vi "get path to CoreEngine dll.vi"() -> (8 "path to wavekit library":path, 12 "Release/Debug":string)   [LabVIEW 2020]
uses:
  <vilib>/registry/registry.llb/Registry RtKey.ctl
  <vilib>/registry/registry.llb/Registry SAM.ctl
  <vilib>/registry/registry.llb/Read Registry Value Simple STR.vi
panel:
  in  "error in (no error)":errorcluster
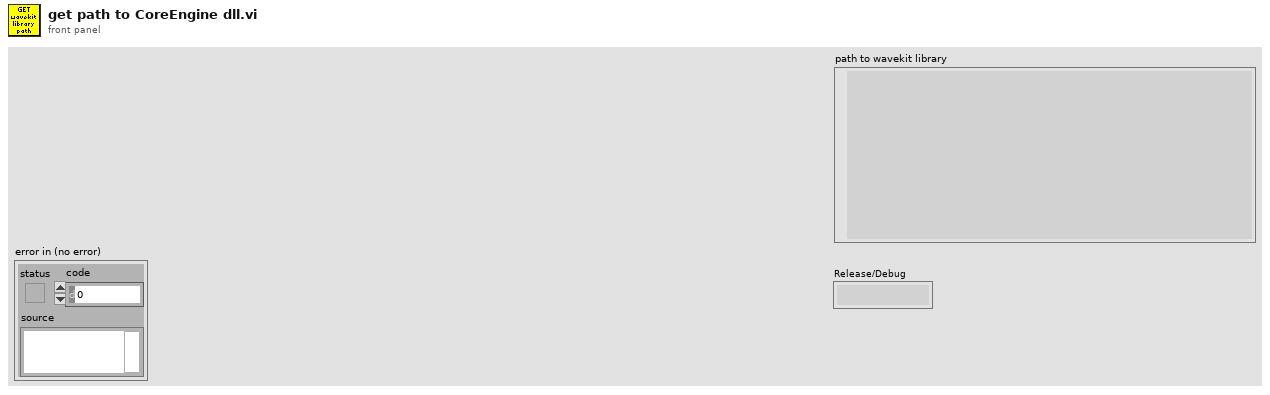
[diagram p1: front panel]
types:
  T1 = typedef "Registry SAM.ctl" = enum32{"KEY_QUERY_VALUE", "KEY_SET_VALUE", "KEY_CREATE_SUB_KEY", "KEY_ENUMERATE_SUB_KEYS", "KEY_NOTIFY", "KEY_CREATE_LINK", "KEY_READ", "KEY_WRITE", "KEY_ALL_ACCESS", "KEY_READ | KEY_WRITE"}
  T2 = typedef "Registry RtKey.ctl" = enum32{"HKEY_CLASSES_ROOT", "HKEY_CURRENT_USER", "HKEY_LOCAL_MACHINE", "HKEY_USERS", "HKEY_PERFORMANCE_DATA", "HKEY_CURRENT_CONFIG", "HKEY_DYN_DATA"}
  T3 = enum32{"invalid app kind", "Development System", "Run Time System", "Student Edition", "Embedded LabVIEW", "Evaluation", "Custom"}
  T4 = typedef "Registry refnum.ctl" = refnum<k1>
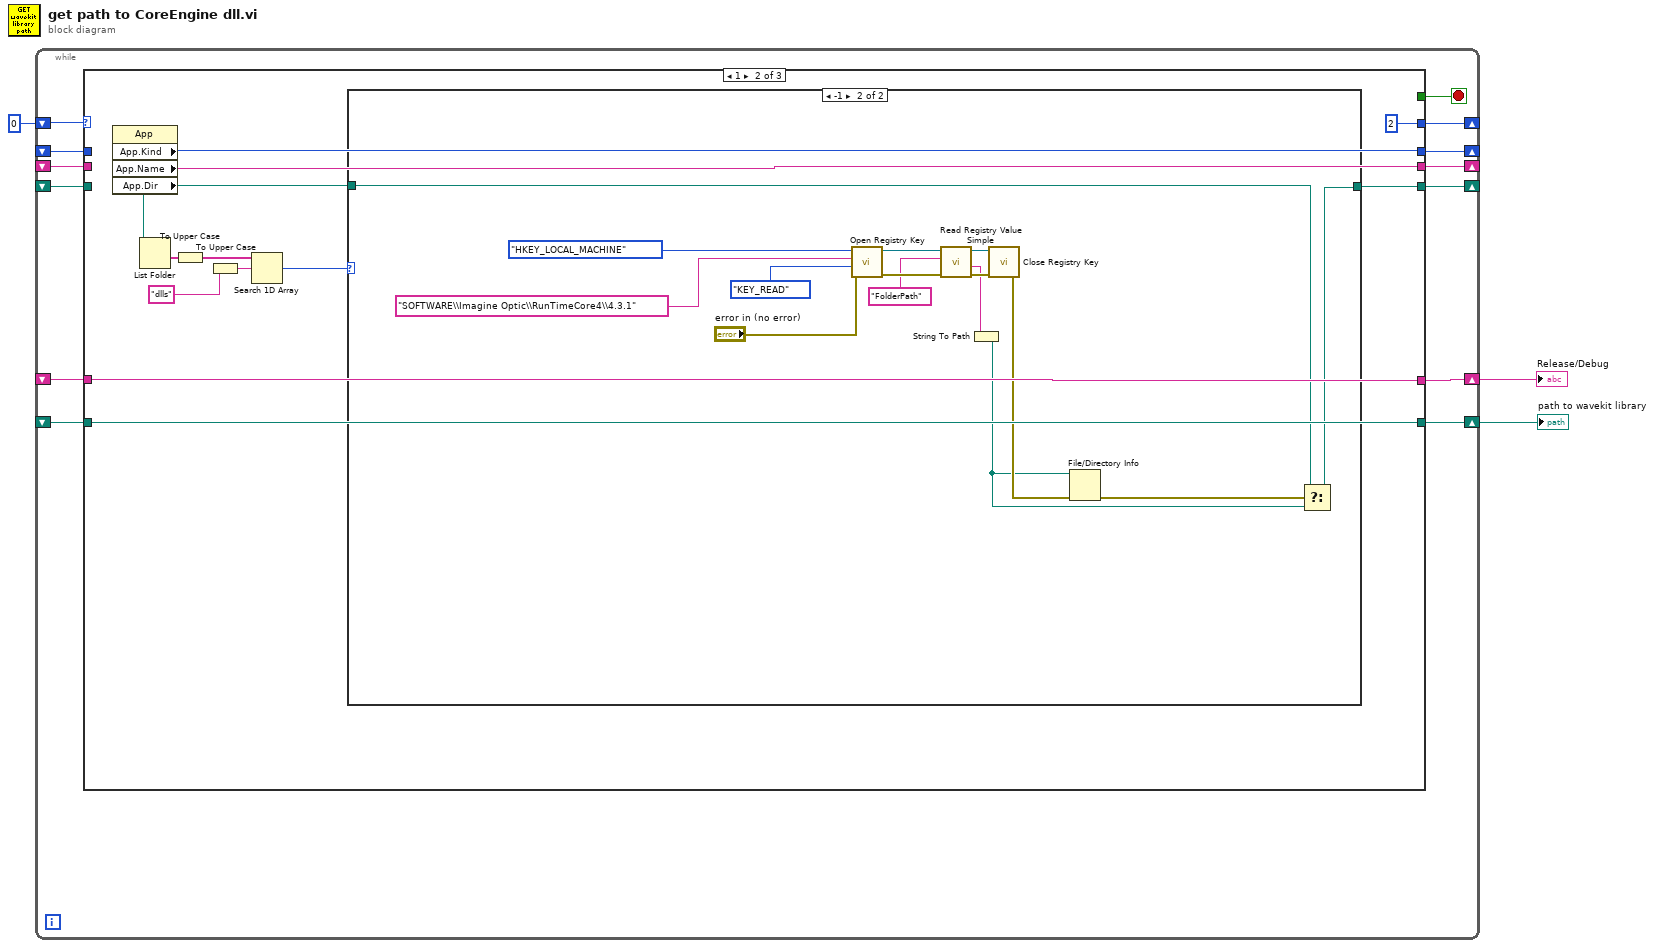
[diagram p0: block diagram]
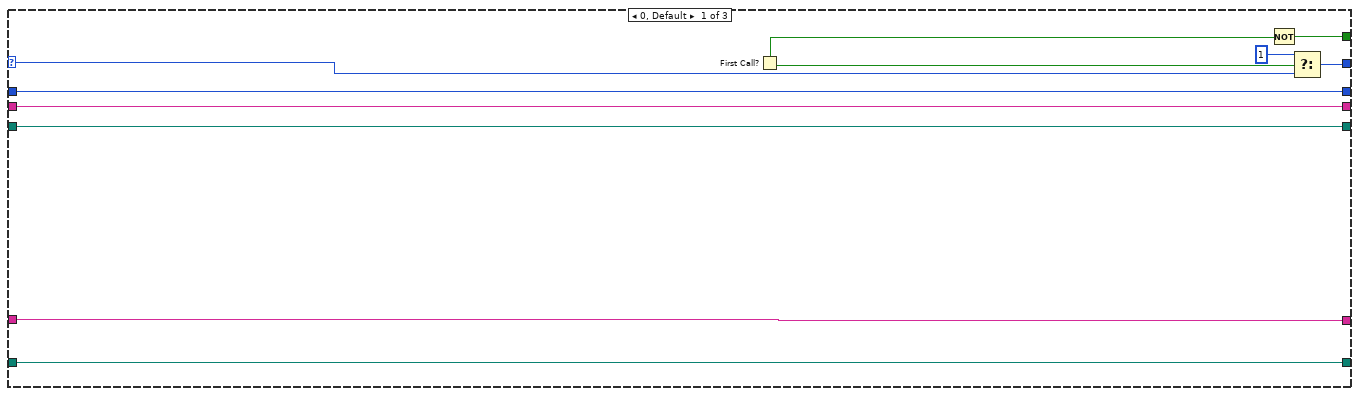
[diagram p2: hidden frame]
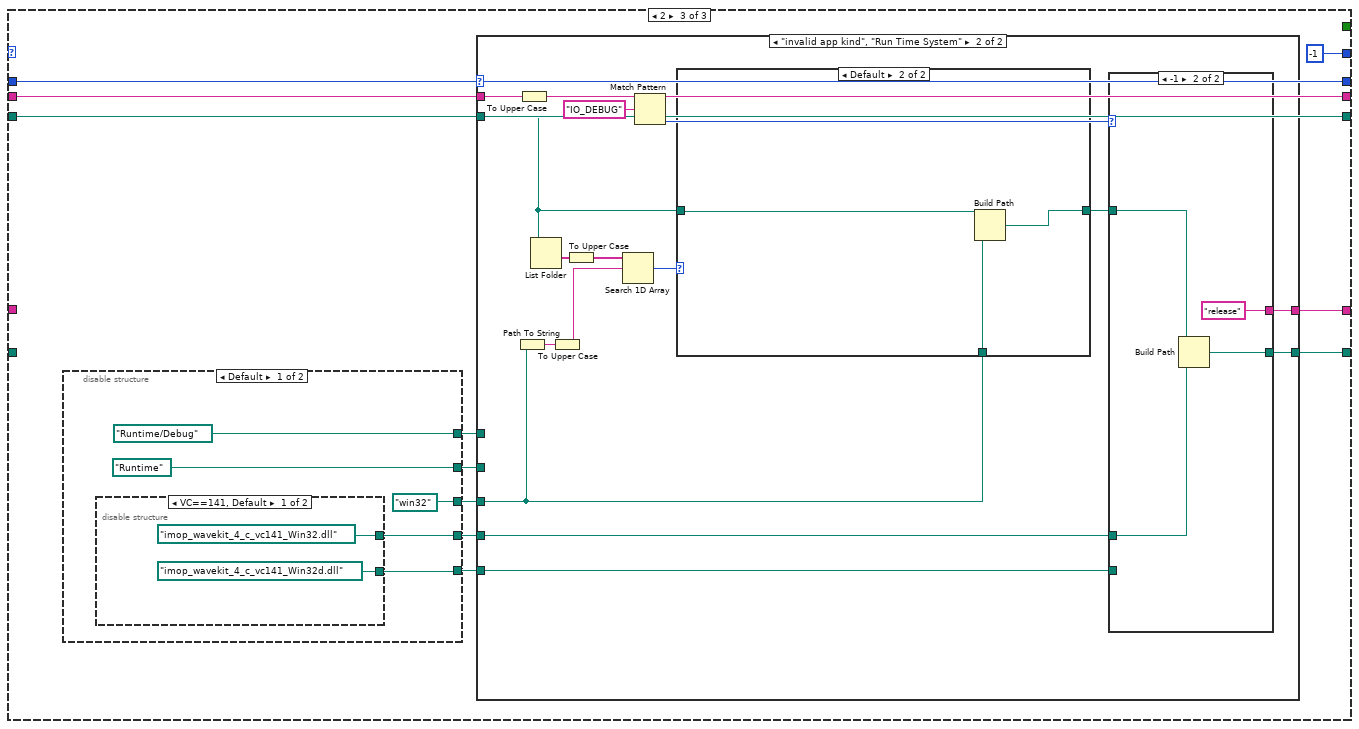
[diagram p4: hidden frame]
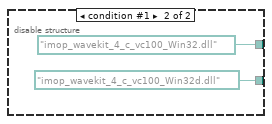
[diagram p5: hidden frame]
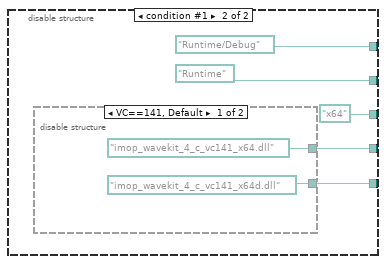
[diagram p6: hidden frame]
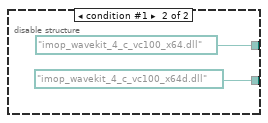
[diagram p7: hidden frame]
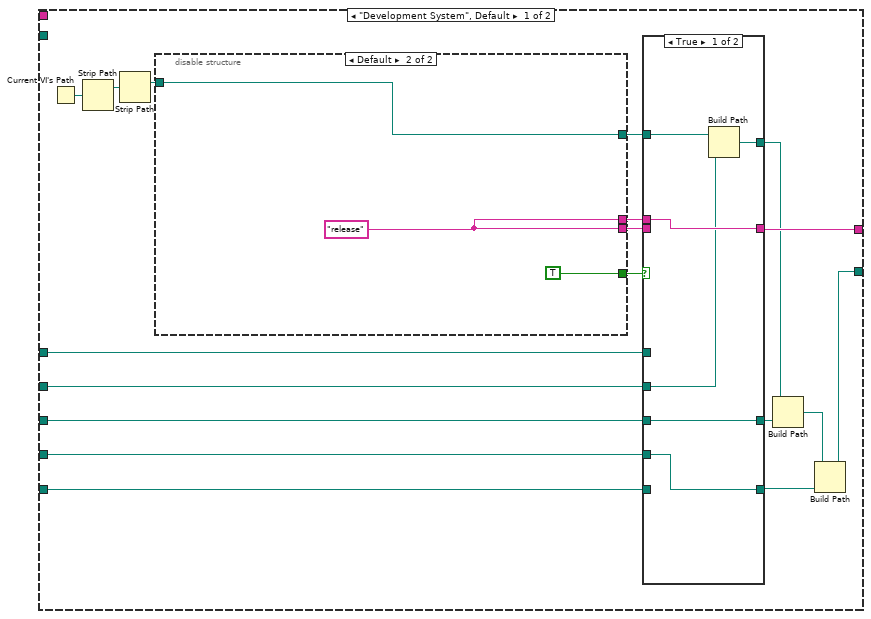
[diagram p8: hidden frame]
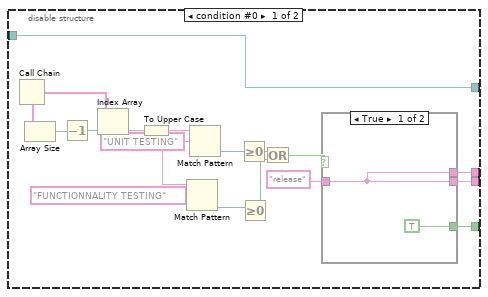
[diagram p9: hidden frame]
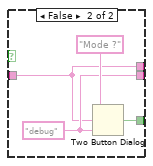
[diagram p10: hidden frame]
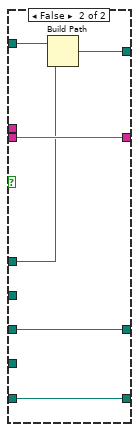
[diagram p11: hidden frame]
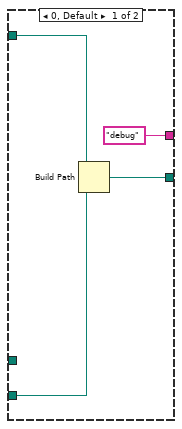
[diagram p12: hidden frame]
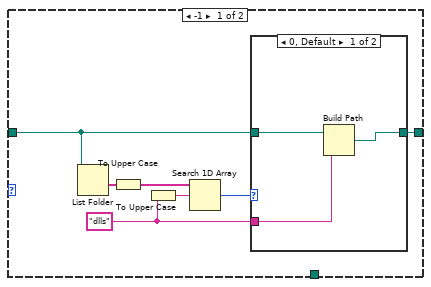
[diagram p13: hidden frame]
diagram:
  n1 = while {
    shift-right: [w14] -> _
    shift-left: 0 -> [w15]
    shift-right: [w12] -> _
    shift-left: _ -> [w9]
    shift-right: [w11] -> _
    shift-left: _ -> [w10]
    shift-right: [w16] -> w3
    shift-left: _ -> [w8]
    shift-right: [w7] -> w1
    shift-left: _ -> [w6]
    shift-right: [w5] -> _
    shift-left: _ -> [w4]
    stop <- w13 stop-if-true
    n2 = case shown="1" w15 {
      selector: w15 -> [w23 _ _]
      tunnel: [w19 w35 w65] -> w16
      tunnel: [w26 2 -1] -> w14
      tunnel: [w22 _ _] -> w13
      tunnel: [w21 w37 w63] -> w12
      tunnel: [w20 w36 w62] -> w11
      tunnel: w10 -> [w20 _ w62]
      tunnel: w9 -> [w21 _ w63]
      tunnel: w8 -> [w19 w35 _]
      tunnel: [w18 w34 w61] -> w7
      tunnel: w6 -> [w18 w34 _]
      tunnel: [w17 w33 w55] -> w5
      tunnel: w4 -> [w17 _ w55]
      frame 0, Default {
        n3 = First Call?() -> (First Call?: T/F=w24:bool)
        n4 = Not(x=w24) -> (.not. x?=w22:bool)
        n5 = Select(t=1, s=w24, f=w23) -> (s? t:f=w26:i32)
      }
      frame 1 {
        n6 = property class="App"() -> ("App.Kind"=w37:T3, "App.Name"=w33:string, "App.Dir"=w28:path)  [unwired: 2 in, 2 out]
        n7 = List Folder(path=w28) -> (folder names=w32:string[])  [unwired: 3 in, 3 out]
        n8 = To Upper Case(1:w32) -> (0:w31:string[])
        n9 = To Upper Case(1:"dlls" ("element")) -> (0:w29:string)
        n10 = Search 1D Array(1D array=w31, element=w29) -> (index of element=w27:i32)  [unwired: 1 in]
        n11 = case shown="-1" w27 {
          tunnel: [w39 w45] -> w36
          tunnel: w28 -> [w39 w42]
          frame 0, Default {
          }
          frame -1 {
            n12 = call <vilib>:"Open Registry Key.vi"("error in (no error)"="error in (no error)", "security access mask (KEY_READ | KEY_WRITE)"=Registry_SAM."KEY_READ", "subkey"="SOFTWARE\\Imagine Optic\\RunTimeCore4\\4.3.1", "root key (HKEY_LOCAL_MACHINE)"=Registry_RtKey."HKEY_LOCAL_MACHINE") -> ("error out"=w52:errorcluster, "refnum out"=w51:T4)  [unwired: 6 in]
            n13 = call-poly <vilib>:"Read Registry Value Simple.vi"("error in (no error)"=w52, "value"="FolderPath", "refnum"=w51) -> ("error out"=w47:errorcluster, "String/Binary data"=w46:string, "refnum out"=w50:T4)  [unwired: 3 in, 1 out]
            n14 = String To Path(string=w46) -> (path=w41:path)
            n15 = call <vilib>:"Close Registry Key.vi"("error in (no error)"=w47, "refnum"=w50) -> ("error out"=w44:errorcluster)  [unwired: 5 in]
            n16 = File/Directory Info(path=w41, error in=w44) -> (error out=w40:errorcluster)  [unwired: 6 out]
            n17 = Select(t=w42, s=w40, f=w41) -> (s? t:f=w45:path)
          }
        }
      }
      frame 2 {
        n18 = disable-structure shown="Default" {
          disable-tunnel: [w68 w79] -> w57
          disable-tunnel: [path "Runtime" ("path in") path "Runtime" ("path in")] -> w59
          disable-tunnel: [path "Runtime/Debug" ("path in") path "Runtime/Debug" ("path in")] -> w60
          disable-tunnel: [w67 w76] -> w56
          disable-tunnel: [path "win32" ("path in") path "x64" ("path in")] -> w58
          frame condition #0 (active) {
            n19 = disable-structure shown="VC==141, Default" {
              disable-tunnel: [path "imop_wavekit_4_c_vc141_Win32.dll" ("path in") path "imop_wavekit_4_c_vc100_Win32.dll" ("path in")] -> w68
              disable-tunnel: [path "imop_wavekit_4_c_vc141_Win32d.dll" ("path in") path "imop_wavekit_4_c_vc100_Win32d.dll" ("path in")] -> w67
              frame condition #0 (active) {
              }
              frame condition #1 {
              }
            }
          }
          frame condition #1 {
            n20 = disable-structure shown="VC==141, Default" {
              disable-tunnel: [path "imop_wavekit_4_c_vc141_x64.dll" ("path in") path "imop_wavekit_4_c_vc100_x64.dll" ("path in")] -> w79
              disable-tunnel: [path "imop_wavekit_4_c_vc141_x64d.dll" ("path in") path "imop_wavekit_4_c_vc100_x64d.dll" ("path in")] -> w76
              frame condition #0 (active) {
              }
              frame condition #1 {
              }
            }
          }
        }
        n21 = case shown="\"invalid app kind\", \"Run Time System\"" w63 {
          tunnel: [w100 w155] -> w61
          tunnel: w62 -> [_ w154]
          tunnel: [w101 w153] -> w65
          tunnel: w57 -> [w99 w146]
          tunnel: w59 -> [w98 _]
          tunnel: w60 -> [w97 _]
          tunnel: w56 -> [w96 w142]
          tunnel: w58 -> [w85 w140]
          tunnel: w55 -> [_ w145]
          frame "Development System", Default {
            n22 = Current VI's Path() -> (path=w91:path)
            n23 = Strip Path(path=w91) -> (stripped path=w92:path)  [unwired: 1 out]
            n24 = Strip Path(path=w92) -> (stripped path=w89:path)  [unwired: 1 out]
            n25 = disable-structure shown="Default" {
              disable-tunnel: [w118 TRUE ("T button?")] -> w95
              disable-tunnel: [w117 w126] -> w94
              disable-tunnel: [w116 w126] -> w93
              disable-tunnel: [w102 w125] -> w90
              disable-tunnel: w89 -> [w102 w125]
              frame condition #0 {
                n26 = Call Chain() -> (call chain=w115:string[])
                n27 = Array Size(array=w115) -> (size(s)=w114:i32)
                n28 = Decrement(x=w114) -> (x-1=w113:i32)
                n29 = Index Array(array=w115, index=w113) -> (element=w112:string)
                n30 = To Upper Case(1:w112) -> (0:w109:string)
                n31 = Match Pattern(string=w109, regular expression="FUNCTIONNALITY TESTING") -> (offset past match=w106:i32)  [unwired: 1 in, 3 out]
                n32 = Match Pattern(string=w109, regular expression="UNIT TESTING") -> (offset past match=w107:i32)  [unwired: 1 in, 3 out]
                n33 = Greater Or Equal To 0?(x=w107) -> (x >= 0?=w105:bool)
                n34 = Greater Or Equal To 0?(x=w106) -> (x >= 0?=w104:bool)
                n35 = Or(x=w105, y=w104) -> (x .or. y?=w103:bool)
                n36 = case shown="True" w103 {
                  tunnel: [TRUE ("T button?") w124] -> w118
                  tunnel: [w120 w121] -> w117
                  tunnel: [w120 w122] -> w116
                  tunnel: "release" ("T button name (\"OK\")") -> [w120 w121]
                  frame True {
                  }
                  frame False {
                    w122 = "debug" ("F button name (\"Cancel\")")
                    n37 = Two Button Dialog(message="Mode ?", 1:w122, 2:w121) -> (T button?=w124:bool)
                  }
                }
              }
              frame condition #1 (active) {
                w126 = "release" ("T button name (\"OK\")")
              }
            }
            n38 = case shown="True" w95 {
              tunnel: [w133 w139] -> w101
              tunnel: w94 -> [w133 _]
              tunnel: w93 -> [_ w139]
              tunnel: w90 -> [w132 w138]
              tunnel: [w131 w137] -> w87
              tunnel: w98 -> [w130 _]
              tunnel: w97 -> [_ w136]
              tunnel: w99 -> [w129 _]
              tunnel: [w129 w135] -> w88
              tunnel: w96 -> [_ w135]
              tunnel: w85 -> [w128 w134]
              tunnel: [w128 w134] -> w84
              frame True {
                n39 = Build Path(base path=w132, name or relative path=w130) -> (appended path=w131:path)
              }
              frame False {
                n40 = Build Path(base path=w138, name or relative path=w136) -> (appended path=w137:path)
              }
            }
            n41 = Build Path(base path=w87, name or relative path=w84) -> (appended path=w86:path)
            n42 = Build Path(base path=w86, name or relative path=w88) -> (appended path=w100:path)
          }
          frame "invalid app kind", "Run Time System" {
            n43 = Path To String(path=w140) -> (string=w148:string)
            n44 = To Upper Case(1:w145) -> (0:w141:string)
            n45 = List Folder(path=w154) -> (folder names=w152:string[])  [unwired: 3 in, 3 out]
            n46 = To Upper Case(1:w148) -> (0:w147:string)
            n47 = To Upper Case(1:w152) -> (0:w151:string[])
            n48 = Search 1D Array(1D array=w151, element=w147) -> (index of element=w150:i32)  [unwired: 1 in]
            n49 = Match Pattern(string=w141, regular expression="IO_DEBUG") -> (offset past match=w143:i32)  [unwired: 1 in, 3 out]
            n50 = case shown="Default" w150 {
              tunnel: [w167 w176] -> w149
              tunnel: w154 -> [w168 w175]
              tunnel: w140 -> [_ w177]
              frame -1 {
                w165 = "dlls" ("element")
                n51 = List Folder(path=w168) -> (folder names=w170:string[])  [unwired: 3 in, 3 out]
                n52 = To Upper Case(1:w170) -> (0:w166:string[])
                n53 = To Upper Case(1:w165) -> (0:w164:string)
                n54 = Search 1D Array(1D array=w166, element=w164) -> (index of element=w169:i32)  [unwired: 1 in]
                n55 = case shown="0, Default" w169 {
                  tunnel: [w171 w174] -> w167
                  tunnel: w168 -> [w173 w174]
                  tunnel: w165 -> [w172 _]
                  frame 0, Default {
                    n56 = Build Path(base path=w173, name or relative path=w172) -> (appended path=w171:path)
                  }
                  frame -1 {
                  }
                }
              }
              frame Default {
                n57 = Build Path(base path=w175, name or relative path=w177) -> (appended path=w176:path)
              }
            }
            n58 = case shown="-1" w143 {
              tunnel: [w159 w163] -> w155
              tunnel: ["debug" ("T button name (\"OK\")") "release" ("T button name (\"OK\")")] -> w153
              tunnel: w149 -> [w157 w161]
              tunnel: w146 -> [_ w160]
              tunnel: w142 -> [w156 _]
              frame 0, Default {
                n59 = Build Path(base path=w157, name or relative path=w156) -> (appended path=w159:path)
              }
              frame -1 {
                n60 = Build Path(base path=w161, name or relative path=w160) -> (appended path=w163:path)
              }
            }
          }
        }
      }
    }
  }
  "path to wavekit library" <- w1
  "Release/Debug" <- w3
